vi "Compressor.vi"(11 "Enum":enum16{"Start", "Run", "End"}(ring)) -> ()   [LabVIEW 2014]
uses:
  <vilib>/Rock Robotics/WPI/Relay/WPI_RelayDirection.ctl
  <vilib>/Rock Robotics/SystemInterfaces/DIO/FPGA_DIORelayChannel.ctl
  <vilib>/Rock Robotics/SystemInterfaces/Typedef/FPGA_TypedefDigitalModule.ctl
  <vilib>/Rock Robotics/SystemInterfaces/DIO/FPGA_DIOChannel.ctl
  <vilib>/Rock Robotics/WPI/Relay/WPI_RelayValue.ctl
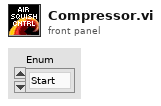
[diagram p1: front panel]
types:
  T1 = typedef "FPGA_DIOChannel.ctl" = enum8{"DIO 1", "DIO 2", "DIO 3", "DIO 4", "DIO 5", "DIO 6", "DIO 7", "DIO 8", "DIO 9", "DIO 10", "DIO 11", "DIO 12", "DIO 13", "DIO 14", "Invalid"}
  T2 = typedef "FPGA_TypedefDigitalModule.ctl" = enum16{"Digital Module 1", "Digital Module 2"}
  T3 = typedef "FPGA_DIORelayChannel.ctl" = enum8{"Relay 1", "Relay 2", "Relay 3", "Relay 4", "Relay 5", "Relay 6", "Relay 7", "Relay 8", "Invalid"}
  T4 = typedef "WPI_RelayDirection.ctl" = enum16{"Both directions", "Forward only", "Reverse only"}
  T5 = typedef "WPI_RelayValue.ctl" = enum16{"Off", "On", "Forward", "Reverse"}
  T6 = typedef "WPI_DigitalInputDevRef.ctl" = cluster{"DevStatus":errorcluster, "DIO Channel":T1, "Digital Module":T2}
  T7 = typedef "WPI_RelayDevRef.ctl" = cluster{"DevStatus":errorcluster, "Relay Channel":T3, "Digital Module":T2, "Relay Direction":T4}
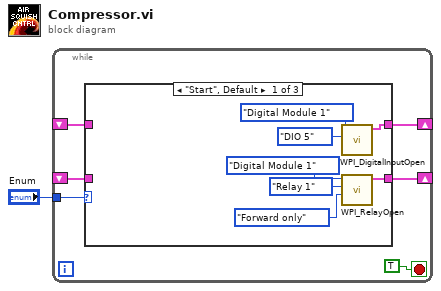
[diagram p0: block diagram]
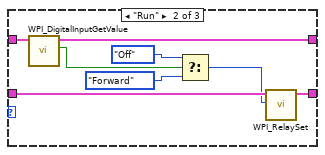
[diagram p2: hidden frame]
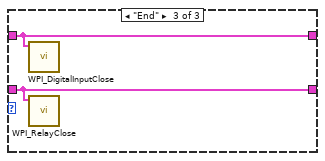
[diagram p3: hidden frame]
diagram:
  n1 = while {
    tunnel: "Enum" -> [w6]
    shift-right: [w4] -> _
    shift-left: _ -> [w5]
    shift-right: [w3] -> _
    shift-left: _ -> [w2]
    stop <- TRUE stop-if-true
    n2 = case shown="\"Start\", Default" w6 {
      tunnel: w5 -> [_ w22 w24]
      tunnel: [w13 w21 w24] -> w4
      tunnel: [w12 w19 w23] -> w3
      tunnel: w2 -> [_ w20 w23]
      frame "Start", Default {
        n3 = call <vilib>:"WPI_DigitalInputOpen.vi"("DIO Channel"=FPGA_DIOChannel."DIO 5", "Digital Module (Module 1)"=FPGA_TypedefDigitalModule."Digital Module 1") -> ("DigitalInputDevRef"=w13:T6)  [unwired: 8 in, 1 out]
        n4 = call <vilib>:"WPI_RelayOpen.vi"("Relay Direction"=WPI_RelayDirection."Forward only", "Relay Channel"=FPGA_DIORelayChannel."Relay 1", "Digital Module (Module 1)"=FPGA_TypedefDigitalModule."Digital Module 1") -> ("RelayDevRef"=w12:T7)  [unwired: 7 in, 1 out]
      }
      frame "Run" {
        n5 = call <vilib>:"WPI_DigitalInputGetValue.vi"("DigitalInputDevRef"=w22) -> ("Value"=w18:bool, "DigitalInputDevRef"=w21:T6)  [unwired: 8 in, 1 out]
        n6 = Select(t=WPI_RelayValue."Off" ("RelayValue"), s=w18, f=WPI_RelayValue."Forward" ("RelayValue")) -> (s? t:f=w15:T5)
        n7 = call <vilib>:"WPI_RelaySet.vi"("RelayValue"=w15, "RelayDevRef"=w20) -> ("RelayDevRef"=w19:T7)  [unwired: 8 in, 1 out]
      }
      frame "End" {
        n8 = call <vilib>:"WPI_DigitalInputClose.vi"("DigitalInputDevRef"=w24) -> ()  [unwired: 10 in, 1 out]
        n9 = call <vilib>:"WPI_RelayClose.vi"("RelayDevRef"=w23) -> ()  [unwired: 10 in, 1 out]
      }
    }
  }
